vi "Convert ASCII to Num Value.vi"(1 "String":string) -> (0 "ASCII Num Value":i32)   [LabVIEW 2012, in "FEM-03.lvlib"]
uses:
  FEM-03.lvlib
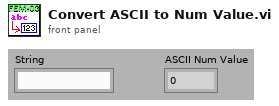
[diagram p1: front panel]
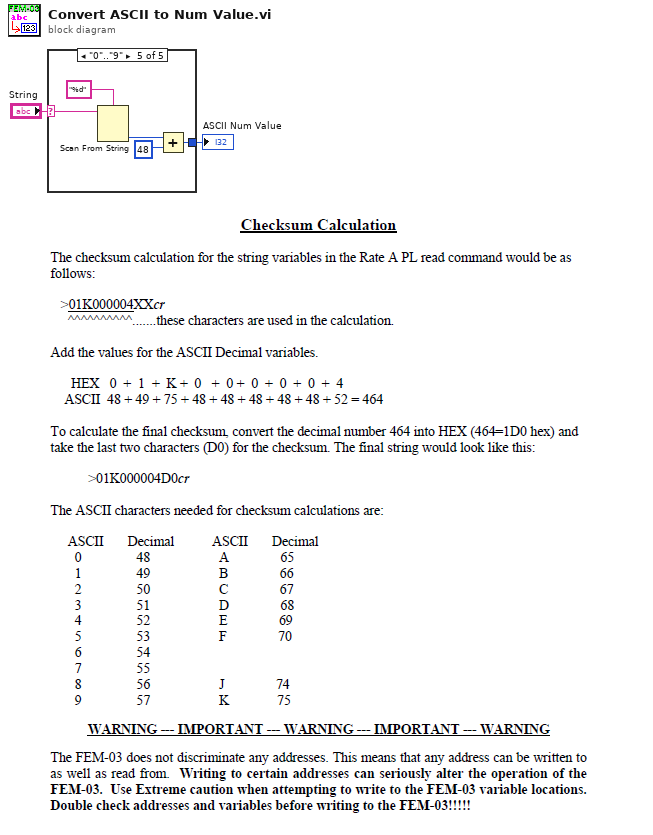
[diagram p0: block diagram]
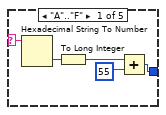
[diagram p2: hidden frame]
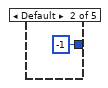
[diagram p3: hidden frame]
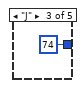
[diagram p4: hidden frame]
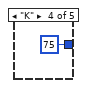
[diagram p5: hidden frame]
diagram:
  n1 = case shown="\"0\"..\"9\"" "String" {
    selector: "String" -> [w7 _ _ _ w15]
    tunnel: [w5 -1 74 75 w11] -> w1
    frame "A".."F" {
      n2 = Hexadecimal String To Number(string=w7) -> (number=w6:u32)  [unwired: 2 in, 1 out]
      n3 = To Long Integer(number=w6) -> (32bit integer=w3:i32)
      n4 = Add(x=w3, y=55) -> (x+y=w5:i32)
    }
    frame Default {
    }
    frame "J" {
    }
    frame "K" {
    }
    frame "0".."9" {
      n5 = Scan From String(format string="%d", input string=w15) -> (output 1=w13:i32)  [unwired: 3 in, 3 out]
      n6 = Add(x=w13, y=48) -> (x+y=w11:i32)
    }
  }
  "ASCII Num Value" <- w1
